vi "Remote.TCP-IP Listener, Convert Function RET to JSON.vi"(8 "Rtn Error":errorcluster, 9 "Data":string[][](array[string])=[["Name1", "Value1"], ["Name2", "Value2"]], 10 "Funct":string="FunctName", 11 "Seq":i32) -> (3 "JSON":string="{\n  \"Seq\":0,\n  \"Funct\":\"FunctionName\",\n  \"Args\":\n        [\n        \"Arg1\",\n        \"Arg2\"\n        ]\n}\n")   [LabVIEW 2024]
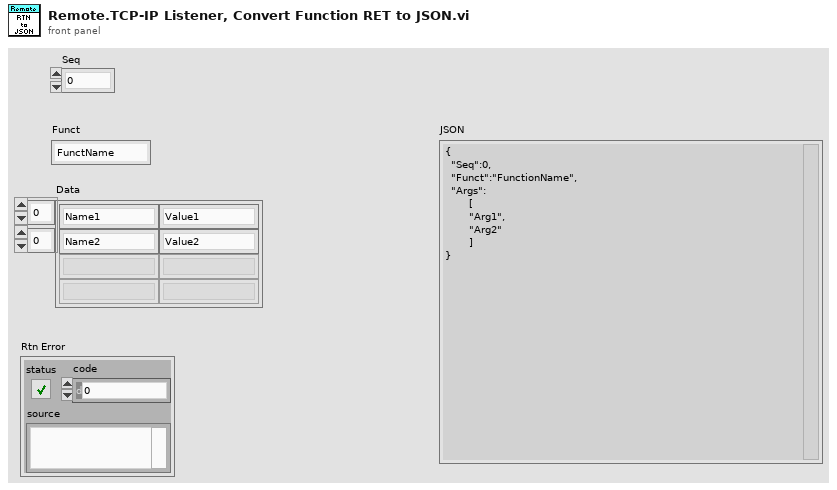
[diagram p1: front panel]
types:
  T1 = cluster{"State":string, "Code":i32, "Desc":string}
  T2 = cluster{"Seq":i32, "Funct":string, "Result":cluster{"State":string, "Code":i32, "Desc":string}, "Data":string[][]}
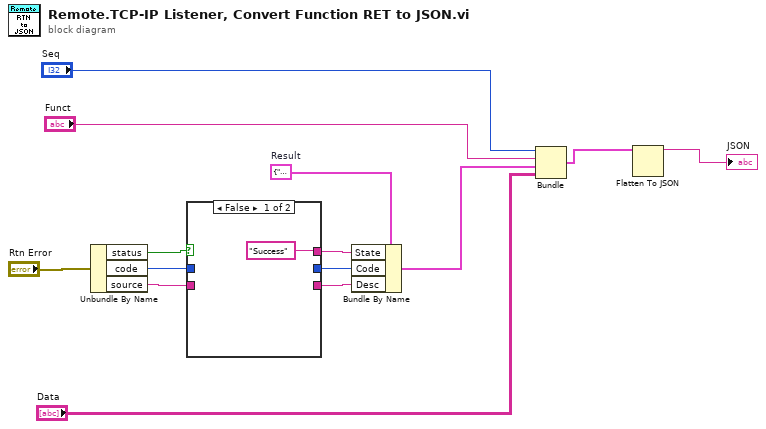
[diagram p0: block diagram]
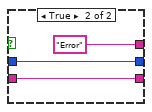
[diagram p2: hidden frame]
diagram:
  w10 = T1 {"State"="", "Code"=0, "Desc"=""}  # Result
  n1 = Unbundle By Name("Rtn Error") -> ("status"=w13:bool, "code"=w12:i32, "source"=w11:string)
  n2 = case shown="False" w13 {
    tunnel: w12 -> [_ w18]
    tunnel: [_ w18] -> w8
    tunnel: w11 -> [_ w16]
    tunnel: ["Success" "Error"] -> w9
    tunnel: [_ w16] -> w7
    frame False {
    }
    frame True {
    }
  }
  n3 = Bundle By Name(cluster=w10, "State"=w9, "Code"=w8, "Desc"=w7) -> (w5:T1)
  n4 = Bundle("Seq"="Seq", "Funct"="Funct", "Result"=w5, "Data"="Data") -> (w2:T2)  [unwired: 1 in]
  n5 = Flatten To JSON(anything=w2) -> (JSON string=→"JSON":string)  [unwired: 2 in, 1 out]
